vi "Matrix_host.vi"() -> ()   [LabVIEW 2018]
uses:
  <vilib>/userdefined/High Color/nirio_resource_hc.ctl
  <vilib>/Utility/error.llb/Error Cluster From Error Code.vi
  <vilib>/rvi/errors/niLvFpgaAdjustHostInterfaceError.vi
  <vilib>/FPGAPlugInAG/Dynamic/niLvFpga_Close_Dynamic.vi
  <vilib>/rvi/interface/nirviReadWriteControl/nirviReadWriteControl.xnode
  <vilib>/rvi/interface/nirviCloseFPGA/nirviCloseFPGA.xnode
  <vilib>/rvi/interface/nirviOpenFPGA/nirviOpenFPGA.xnode
  <vilib>/rvi/interface/nirviMethod/nirviMethod.xnode
  FPGA Bitfiles/Matrix_FPGATarget_Matrixtarget_hwzlcigaD4Q.lvbitx
  NiFpgaLv.dll
  <vilib>/rvi/interface/Simulation/niFpgaSimulationCallBeginRW.vi
  <vilib>/FPGAPlugInAG/Dynamic/niLvFpga_Reset_Dynamic.vi
  <vilib>/FPGAPlugInAG/Dynamic/niLvFpga_Run_Dynamic.vi
  <vilib>/FPGAPlugInAG/PXI-7953R/niLvFpga_Open_PXI-7953R.vi
  <vilib>/rvi/interface/common/dynamic/niFpgaDynamicAddResources.vi
panel:
  out "ArrayUp":u64
  out "ArrayLow":u64
  in  "DataLow":u8 format="%x"
  in  "Device":u8 format="%x"
  in  "DataUp":u8 format="%x"
  in  "Reg":u8 format="%x"
  in  "Send":bool=TRUE
  in  "ПЛИС":T1
  in  "Стоп":bool
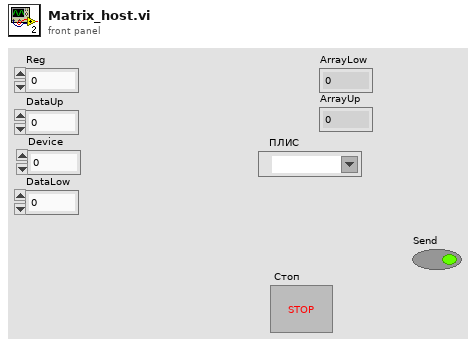
[diagram p1: front panel]
types:
  T1 = typedef "nirio_resource_hc.ctl" = tag
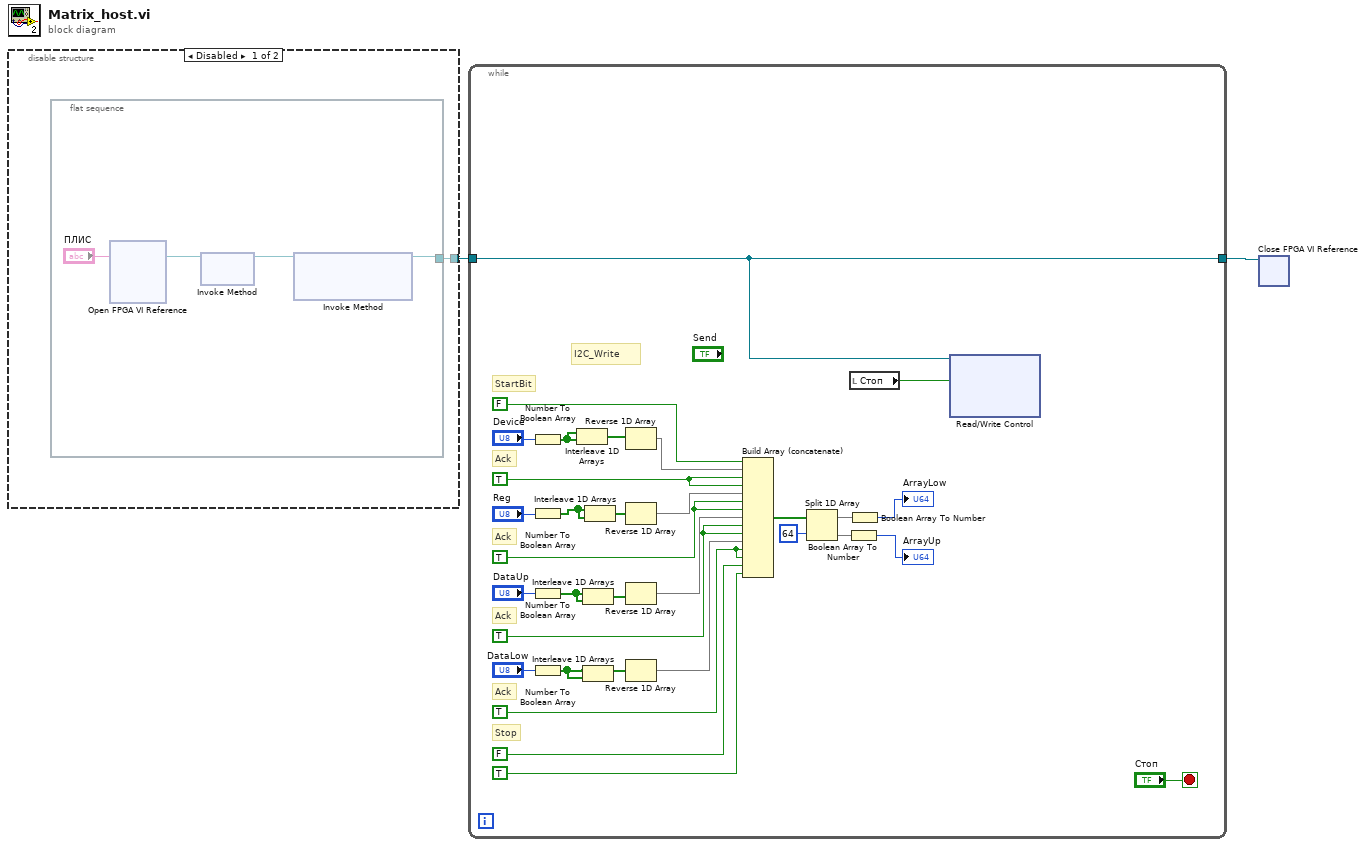
[diagram p0: block diagram]
diagram:
  n1 = disable-structure shown="Disabled" {
    disable-tunnel: [w3 _] -> w2
    frame Disabled {
      n2 = flat-sequence {
        tunnel: [w7] -> w3
        frame #0 {
          n3 = xnode "Open FPGA VI Reference"("resource name"="ПЛИС") -> ("FPGA VI Reference Out"=w5:refnum<k20>)  [unwired: 1 in, 1 out]
          n4 = xnode "Invoke Method"("FPGA VI Reference In"=w5) -> ("FPGA VI Reference Out"=w4:refnum<k20>)  [unwired: 1 in, 1 out]
          n5 = xnode "Invoke Method"("FPGA VI Reference In"=w4) -> ("FPGA VI Reference Out"=w7:refnum<k20>)  [unwired: 2 in, 1 out]
        }
      }
    }
    frame Enabled {
    }
  }
  n6 = while {
    tunnel: w2 -> [w38]
    tunnel: [w38] -> w1
    stop <- "Стоп" stop-if-true
    w24 = TRUE
    w27 = TRUE
    w30 = TRUE
    w33 = TRUE
    # "Stop"
    # "Ack"
    # "Ack"
    # "Ack"
    # "Ack"
    # "StartBit"
    # "I2C_Write"
    n7 = Number To Boolean Array(number="Device") -> (Boolean array=w21:bool[])
    n8 = Number To Boolean Array(number="Reg") -> (Boolean array=w15:bool[])
    n9 = Number To Boolean Array(number="DataUp") -> (Boolean array=w16:bool[])
    n10 = Number To Boolean Array(number="DataLow") -> (Boolean array=w14:bool[])
    n11 = Interleave 1D Arrays(w21, w21) -> (w20:bool[])
    n12 = Interleave 1D Arrays(w16, w16) -> (w17:bool[])
    n13 = Interleave 1D Arrays(w14, w14) -> (w19:bool[])
    n14 = Interleave 1D Arrays(w15, w15) -> (w18:bool[])
    n15 = Reverse 1D Array(array=w20) -> (reversed array=w35:bool[])
    n16 = Reverse 1D Array(array=w18) -> (reversed array=w32:bool[])
    n17 = Reverse 1D Array(array=w17) -> (reversed array=w28:bool[])
    n18 = Reverse 1D Array(array=w19) -> (reversed array=w26:bool[])
    n19 = Build Array (concatenate)(FALSE, w35, w33, w33, w32, w30, w30, w28, w27, w27, w26, w24, w24, FALSE, TRUE) -> (w10:bool[])
    n20 = Split 1D Array(array=w10, index=u64 64) -> (first subarray=w9:bool[], second subarray=w8:bool[])
    n21 = Boolean Array To Number(Boolean array=w8) -> (number=→"ArrayUp":u64)
    n22 = local read "Стоп"() -> (w37:bool)
    n23 = Boolean Array To Number(Boolean array=w9) -> (number=→"ArrayLow":u64)
    n24 = xnode "Read/Write Control"("FPGA VI Reference In"=w38, "Стоп"=w37) -> ()  [unwired: 2 in, 3 out]
  }
  n25 = xnode "Close FPGA VI Reference"("FPGA VI Reference In"=w1) -> ()  [unwired: 1 in, 1 out]
